vi "Find Item in ProjectItem.vi"(7 "Type":string, 8 "error in (no error)":errorcluster, 10 "Item Name":string, 11 "ProjectItem in":refnum<vi>) -> (0 "error out":errorcluster, 1 "Found ?":bool, 2 "Item out":refnum<vi>, 3 "ProjectItem out":refnum<vi>)   [LabVIEW 2019, in "Project Sync Tools.lvclass"]
uses:
  Project Sync Tools.lvclass
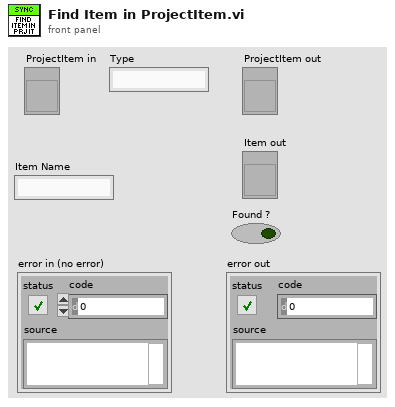
[diagram p1: front panel]
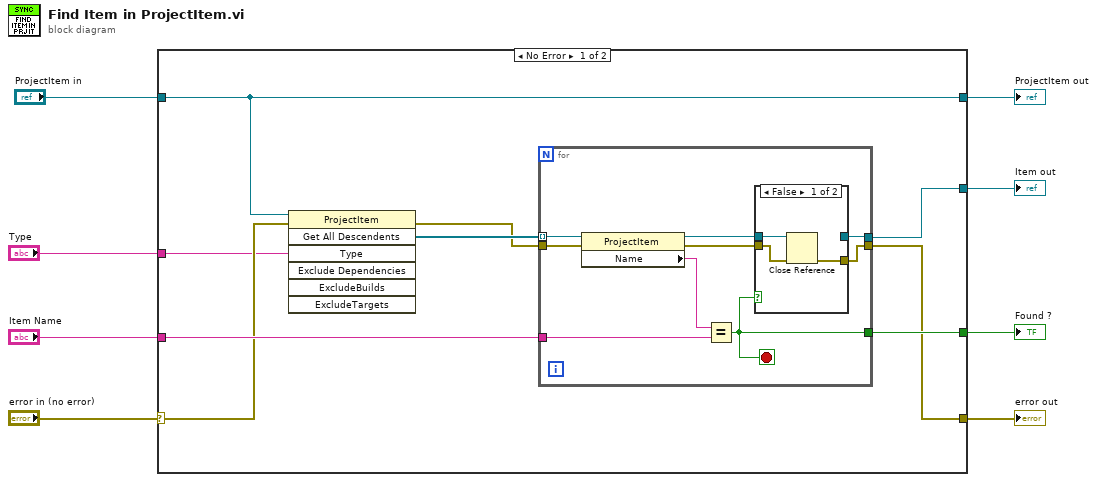
[diagram p0: block diagram]
diagram:
  n1 = case shown="No Error" "error in (no error)" {
    selector: "error in (no error)" -> [w12 w33]
    tunnel: [w17 _] -> w8
    tunnel: [w16 _] -> w7
    tunnel: "Item Name" -> [w14 _]
    tunnel: [w13 w33] -> w5
    tunnel: "Type" -> [w11 _]
    tunnel: "ProjectItem in" -> [w10 w32]
    tunnel: [w10 w32] -> w1
    frame No Error {
      n2 = invoke class="ProjectItem" method="Get All Descendents"(reference=w10, error in=w12, "Type"=w11) -> (error out=w9:errorcluster, "All Descendents"=w15:refnum<vi>[])  [unwired: 4 in, 5 out]
      n3 = for {
        tunnel: w15 -> [w26] mode=indexing
        tunnel: w14 -> [w25]
        tunnel: [w20] -> w13
        tunnel: [w23] -> w16
        tunnel: [w19] -> w17
        tunnel: w9 -> [w18]
        stop <- w23 stop-if-true
        n4 = property class="ProjectItem"(reference=w26, error in=w18) -> (reference out=w22:refnum<vi>, error out=w21:errorcluster, "Name"=w24:string)
        n5 = Equal?(x=w24, y=w25) -> (x = y?=w23:bool)
        n6 = case shown="False" w23 {
          tunnel: w22 -> [w29 w31]
          tunnel: w21 -> [w28 w30]
          tunnel: [w27 w30] -> w20
          tunnel: [_ w31] -> w19
          frame False {
            n7 = Close Reference(reference=w29, error in (no error)=w28) -> (error out=w27:errorcluster)
          }
          frame True {
          }
        }
      }
    }
    frame Error {
    }
  }
  "Item out" <- w8
  "Found ?" <- w7
  "error out" <- w5
  "ProjectItem out" <- w1
